vi "Generate_WayPoints_ConstantDistanceNOREVERSE.vi"(5 "Update Position Loop Wait Time (us)":u32=50000, 11 "Input Cluster":T2={"Scan Rate (um/s)"=15.0, "X Start"=15.0, "X End"=15.0, "Y Start"=15.0, "Y End"=15.0, " Z Start"=15.0, "Number of Lines"=15, "V"=15.0, "Z End"=15.0, "Approach Rate (um/s)"=15.0, "HoldTime / s"=15}) -> (0 "output cluster":T1)   [LabVIEW 2023]
uses:
  TypeDefs/WayPointCluster.ctl
  User_Vi/Settings.vi
panel:
  out "X Current":dbl
  in  "WayPointCluster":T1
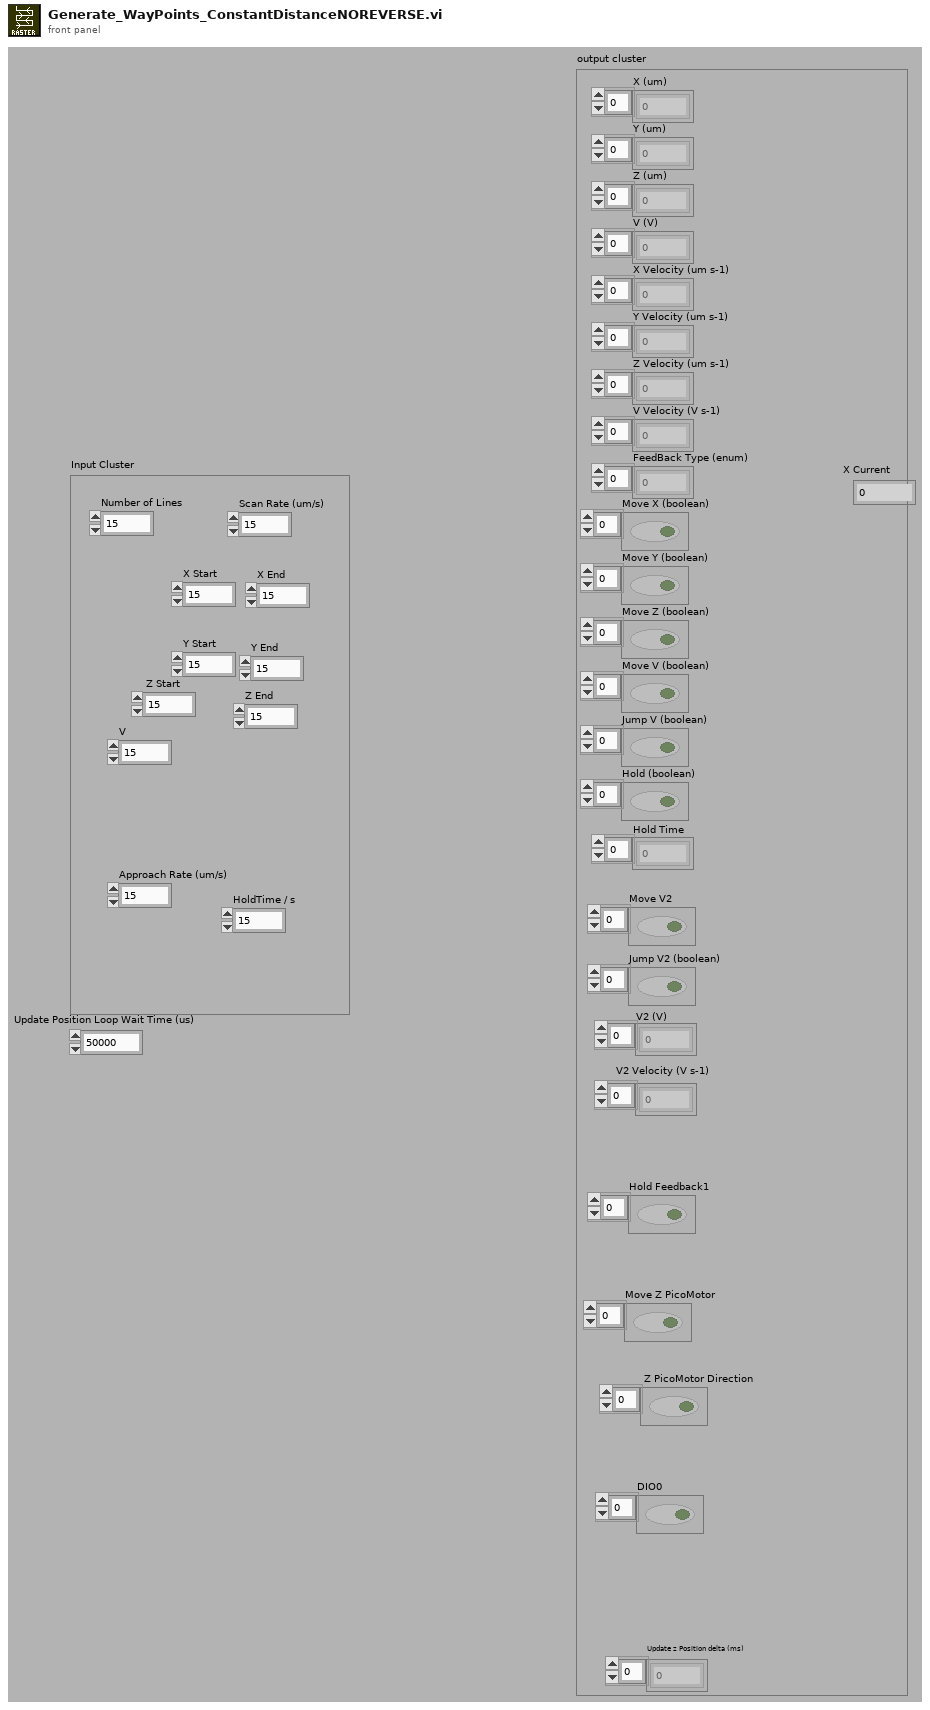
[diagram p1: front panel]
types:
  T1 = typedef "WayPointCluster.ctl" = cluster{"X (um)":dbl[], "Y (um)":dbl[], "Z (um)":dbl[], "V (V)":dbl[], "X Velocity (um s-1)":dbl[], "Y Velocity (um s-1)":dbl[], "Z Velocity (um s-1)":dbl[], "V Velocity (V s-1)":dbl[], "FeedBack Type (enum)":u16[], "Move X (boolean)":bool[], "Move Y (boolean)":bool[], "Move Z (boolean)":bool[], "Move V (boolean)":bool[], "Jump V (boolean)":bool[], "Hold (boolean)":bool[], "Hold Time":u32[], "V2 (V)":dbl[], "Move V2":bool[], "V2 Velocity (V s-1)":dbl[], "Jump V2 (boolean)":bool[], "Update z Position delta (ms)":i16[], "Hold Feedback1":bool[], "Move Z PicoMotor":bool[], " Z PicoMotor Direction":bool[], "DIO0":bool[]}
  T2 = cluster{"Scan Rate (um/s)":dbl, "X Start":dbl, "X End":dbl, "Y Start":dbl, "Y End":dbl, " Z Start":dbl, "Number of Lines":u32, "V":dbl, "Z End":dbl, "Approach Rate (um/s)":dbl, "HoldTime / s":u32}
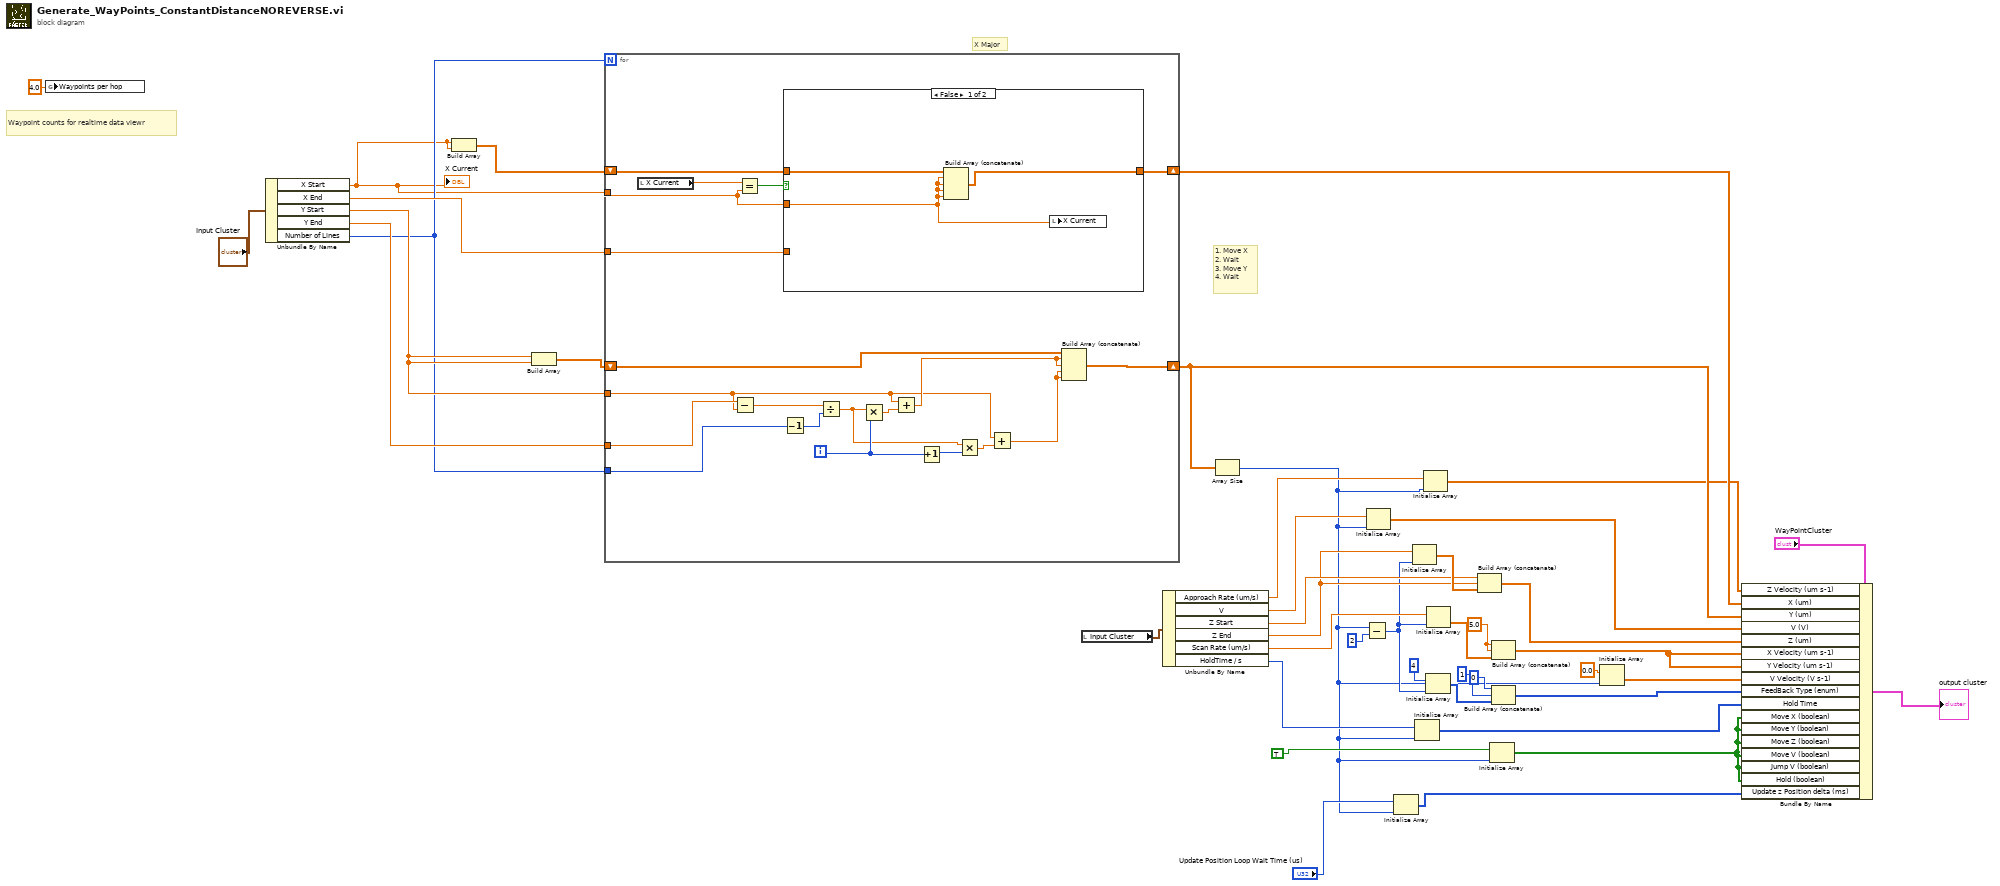
[diagram p0: block diagram]
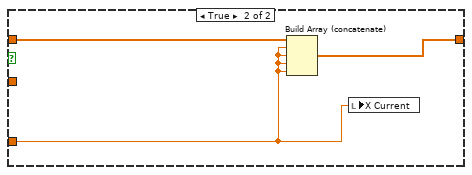
[diagram p2: hidden frame]
diagram:
  w27 = 5.0 ("element")
  # "Waypoint counts for realtime data viewr"
  # "1. Move X\n2. Wait\n3. Move Y\n4. Wait"
  # "X Major"
  n1 = global write "Settings.vi" "Waypoints per hop"(4.0 ("Waypoints per hop")) -> ()
  n2 = Unbundle By Name("Input Cluster") -> ("X Start"=w7:dbl, "X End"=w10:dbl, "Y Start"=w9:dbl, "Y End"=w41:dbl, "Number of Lines"=w8:u32)
  "X Current" <- w7
  n3 = Build Array(w7, w7) -> (w11:dbl[])
  n4 = Build Array(w9, w9) -> (w12:dbl[])
  n5 = for {
    N: w8 -> [_]
    tunnel: w41 -> [w62]
    tunnel: w8 -> [w59]
    shift-right: [w54] -> w6
    shift-left: w12 -> [w58]
    shift-right: [w55] -> w40
    shift-left: w11 -> [w57]
    tunnel: w10 -> [w53]
    tunnel: w9 -> [w45]
    tunnel: w7 -> [w43]
    i -> [w49]
    n6 = local read "X Current"() -> (w50:dbl)
    n7 = Subtract(x=w62, y=w45) -> (x-y=w61:dbl)
    n8 = Equal?(x=w50, y=w43) -> (x = y?=w51:bool)
    n9 = case shown="False" w51 {
      tunnel: w57 -> [w64 w68]
      tunnel: [w65 w67] -> w55
      tunnel: w53 -> [_ w66]
      tunnel: w43 -> [w63 _]
      frame False {
        n10 = Build Array (concatenate)(w64, w63, w63, w63, w63) -> (w65:dbl[])
        n11 = local write "X Current"(w63) -> ()
      }
      frame True {
        n12 = Build Array (concatenate)(w68, w66, w66, w66, w66) -> (w67:dbl[])
        n13 = local write "X Current"(w66) -> ()
      }
    }
    n14 = Decrement(x=w59) -> (x-1=w56:u32)
    n15 = Divide(x=w61, y=w56) -> (x/y=w46:dbl)
    n16 = Multiply(x=w46, y=w49) -> (x*y=w60:dbl)
    n17 = Add(x=w45, y=w60) -> (x+y=w52:dbl)
    n18 = Increment(x=w49) -> (x+1=w47:i32)
    n19 = Multiply(x=w46, y=w47) -> (x*y=w48:dbl)
    n20 = Add(x=w45, y=w48) -> (x+y=w44:dbl)
    n21 = Build Array (concatenate)(w58, w52, w52, w44, w44) -> (w54:dbl[])
  }
  n22 = local read "Input Cluster"() -> (w38:T2)
  n23 = Unbundle By Name(w38) -> ("Approach Rate (um/s)"=w4:dbl, "V"=w16:dbl, "Z Start"=w19:dbl, "Z End"=w18:dbl, "Scan Rate (um/s)"=w31:dbl, "HoldTime / s"=w37:u32)
  n24 = Array Size(array=w6) -> (size(s)=w3:i32)
  n25 = Subtract(x=w3, y=2) -> (x-y=w5:i32)
  n26 = Initialize Array(w16, w3) -> (w15:dbl[])
  n27 = Initialize Array("Update Position Loop Wait Time (us)", w3) -> (w13:u32[])
  n28 = Initialize Array(w18, w5) -> (w20:dbl[])
  n29 = Initialize Array(w37, w3) -> (w32:u32[])
  n30 = Initialize Array(w4, w3) -> (w2:dbl[])
  n31 = Initialize Array(u32 4 ("element"), w5) -> (w23:u32[])
  n32 = Initialize Array(w31, w5) -> (w28:dbl[])
  n33 = Build Array (concatenate)(w19, w18, w20) -> (w17:dbl[])
  n34 = Initialize Array(TRUE, w3) -> (w21:bool[])
  n35 = Build Array (concatenate)(w27, w27, w28) -> (w29:dbl[])
  n36 = Build Array (concatenate)(u32 0 ("element"), u32 1 ("element"), w23) -> (w22:u32[])
  n37 = Initialize Array(0.0 ("element"), w3) -> (w33:dbl[])
  n38 = Bundle By Name(cluster="WayPointCluster", "Z Velocity (um s-1)"=w2, "X (um)"=w40, "Y (um)"=w6, "V (V)"=w15, "Z (um)"=w17, "X Velocity (um s-1)"=w29, "Y Velocity (um s-1)"=w29, "V Velocity (V s-1)"=w33, "FeedBack Type (enum)"=w22, "Hold Time"=w32, "Move X (boolean)"=w21, "Move Y (boolean)"=w21, "Move Z (boolean)"=w21, "Move V (boolean)"=w21, "Jump V (boolean)"=w21, "Hold (boolean)"=w21, "Update z Position delta (ms)"=w13) -> (→"output cluster":T1)
